vi "Datatypes.vi"() -> ()   [LabVIEW 2019]
panel:
  out "Integer out":i32
  out "Boolean out":bool
  out "Floating Point out":dbl
  out "String out":string
  out "File Path out":path
  out "Waveform Chart":dbl(graph)
  in  "File Path":path
  in  "String":string
  in  "Floating Point":dbl
  in  "Boolean":bool
  in  "Integer":i32
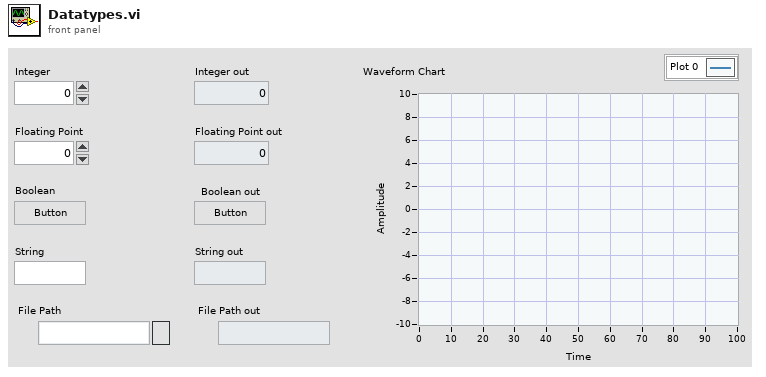
[diagram p1: front panel]
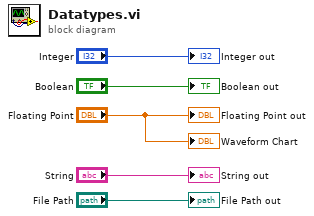
[diagram p0: block diagram]
diagram:
  "Waveform Chart" <- "Floating Point"
  "File Path out" <- "File Path"
  "String out" <- "String"
  "Floating Point out" <- "Floating Point"
  "Boolean out" <- "Boolean"
  "Integer out" <- "Integer"
